vi "test-translation2d.vi"() -> ()   [LabVIEW 2019]
uses:
  <vilib>/Rock Robotics/WPI/ThirdParty/JAS_Junk/TrajLib/Util_CalcDist.vi
  <vilib>/Rock Robotics/WPI/ThirdParty/JAS_Junk/TrajLib/Trajectory_Library.lvlib
panel:
  out "T7 -- y -- 0":dbl
  out "T7 -- X -- 0":dbl
  out "T6 -- dist - 0":dbl
  out "T5 -- norm - 0":dbl
  out "T4 -- y -- 0":dbl
  out "T4 -- X -- 0":dbl
  out "T3 -- y -- 0":dbl
  out "T3 -- X -- 0":dbl
  out "T2 -- y -- 0":dbl
  out "T2 -- X -- 0":dbl
  out "T9 - False":bool
  out "T8 - True":bool
  out "T1 -- y -- 0":dbl
  out "T1 -- X -- 0":dbl
  out "T0 -- y -- 0":dbl
  out "T0 -- X -- 0":dbl
  # "Translation2D Test"
  # "Didn't implement divide"
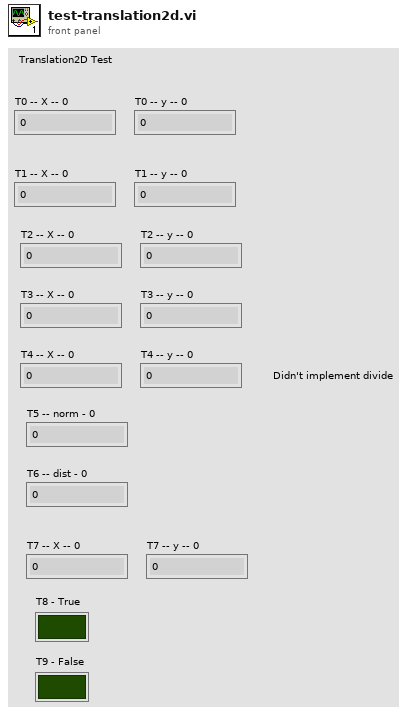
[diagram p1: front panel]
types:
  T1 = typedef "Trajectory_Library.lvlib/TRANSLATION2D.ctl" = cluster{"X":dbl, "Y":dbl}
  T2 = typedef "Trajectory_Library.lvlib/ROTATION2D.ctl" = cluster{"VALUE":dbl, "COS":dbl, "SIN":dbl}
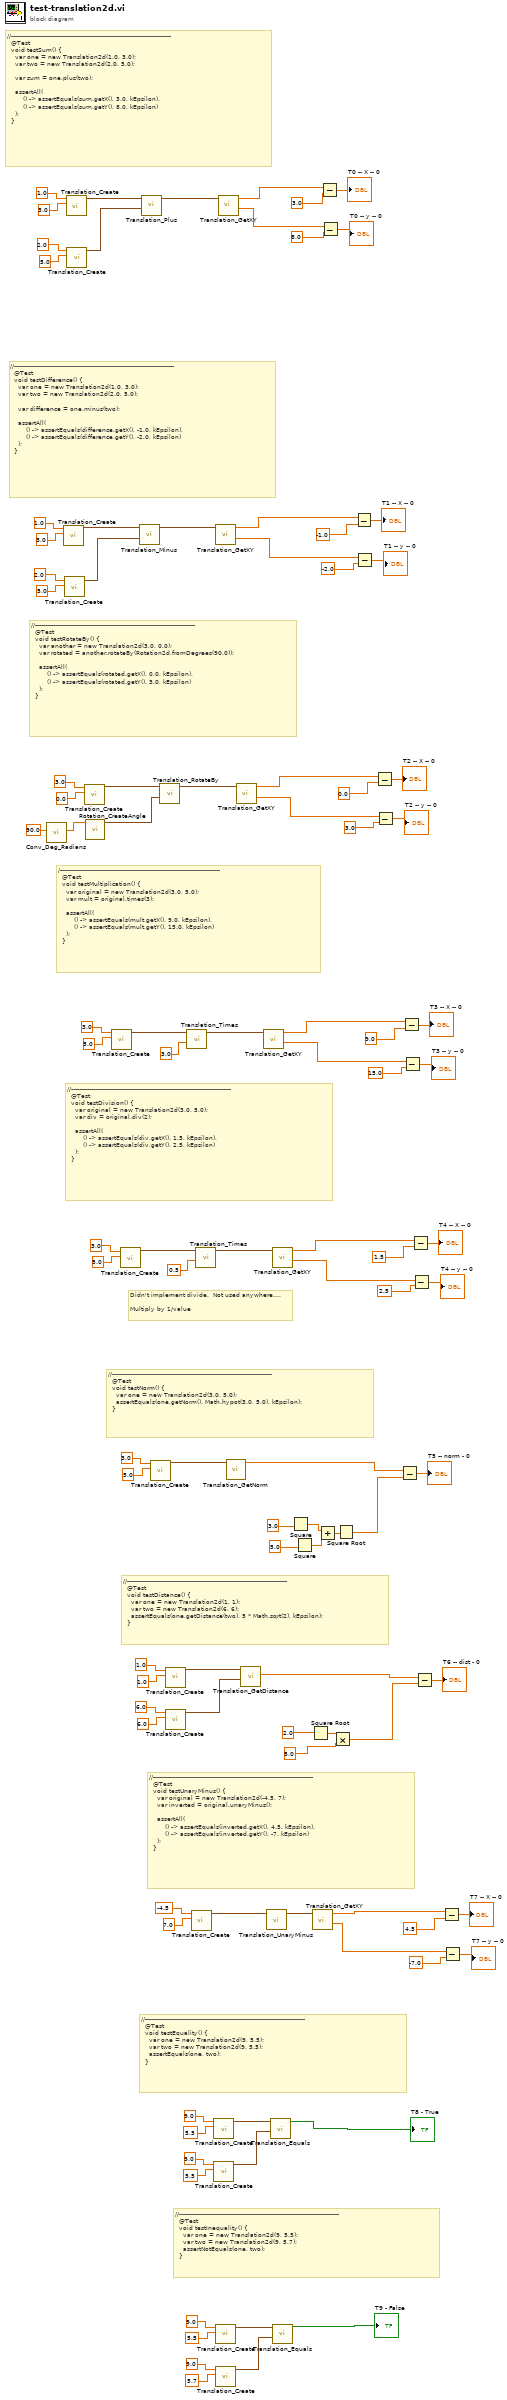
[diagram p0: block diagram]
diagram:
  # "//--------------------------------------------------------------------------------\n  @Test\n  void testInequality() {\n    var one = new Translation2d(9, 5.5);\n    var two = new Translation2d(9, 5.7);\n    assertNotEquals(one, two);\n  }"
  # "//--------------------------------------------------------------------------------\n  @Test\n  void testUnaryMinus() {\n    var original = new Translation2d(-4.5, 7);\n    var inverted = original.unaryMinus();\n\n    assertAll(\n        () -> assertEquals(inverted.getX(), 4.5, kEpsilon),\n        () -> assertEquals(inverted.getY(), -7, kEpsilon)\n    );\n  }"
  # "//--------------------------------------------------------------------------------\n  @Test\n  void testDistance() {\n    var one = new Translation2d(1, 1);\n    var two = new Translation2d(6, 6);\n    assertEquals(one.getDistance(two), 5 * Math.sqrt(2), kEpsilon);\n  }"
  # "//--------------------------------------------------------------------------------\n  @Test\n  void testNorm() {\n    var one = new Translation2d(3.0, 5.0);\n    assertEquals(one.getNorm(), Math.hypot(3.0, 5.0), kEpsilon);\n  }"
  # "Didn't implement divide.  Not used anywhere....\n\nMultiply by 1/value"
  # "//--------------------------------------------------------------------------------\n  @Test\n  void testDivision() {\n    var original = new Translation2d(3.0, 5.0);\n    var div = original.div(2);\n\n    assertAll(\n        () -> assertEquals(div.getX(), 1.5, kEpsilon),\n        () -> assertEquals(div.getY(), 2.5, kEpsilon)\n    );\n  }"
  # "/--------------------------------------------------------------------------------\n  @Test\n  void testMultiplication() {\n    var original = new Translation2d(3.0, 5.0);\n    var mult = original.times(3);\n\n    assertAll(\n        () -> assertEquals(mult.getX(), 9.0, kEpsilon),\n        () -> assertEquals(mult.getY(), 15.0, kEpsilon)\n    );\n  }"
  # "//--------------------------------------------------------------------------------\n  @Test\n  void testRotateBy() {\n    var another = new Translation2d(3.0, 0.0);\n    var rotated = another.rotateBy(Rotation2d.fromDegrees(90.0));\n\n    assertAll(\n        () -> assertEquals(rotated.getX(), 0.0, kEpsilon),\n        () -> assertEquals(rotated.getY(), 3.0, kEpsilon)\n    );\n  }"
  # "//--------------------------------------------------------------------------------\n  @Test\n  void testEquality() {\n    var one = new Translation2d(9, 5.5);\n    var two = new Translation2d(9, 5.5);\n    assertEquals(one, two);\n  }"
  # "//--------------------------------------------------------------------------------\n  @Test\n  void testDifference() {\n    var one = new Translation2d(1.0, 3.0);\n    var two = new Translation2d(2.0, 5.0);\n\n    var difference = one.minus(two);\n\n    assertAll(\n        () -> assertEquals(difference.getX(), -1.0, kEpsilon),\n        () -> assertEquals(difference.getY(), -2.0, kEpsilon)\n    );\n  }"
  # "//--------------------------------------------------------------------------------\n  @Test\n  void testSum() {\n    var one = new Translation2d(1.0, 3.0);\n    var two = new Translation2d(2.0, 5.0);\n\n    var sum = one.plus(two);\n\n    assertAll(\n        () -> assertEquals(sum.getX(), 3.0, kEpsilon),\n        () -> assertEquals(sum.getY(), 8.0, kEpsilon)\n    );\n  }"
  n1 = call <vilib>:"Conv_Deg_Radians.vi"("Degress"=90.0) -> ("Radians"=w72:dbl)  [unwired: 10 in]
  n2 = call <vilib>:"Translation_Create.vi"("Y"=3.0, "X"=1.0) -> ("TRANSLATION"=w88:T1)  [unwired: 9 in]
  n3 = call <vilib>:"Translation_Create.vi"("Y"=5.0, "X"=2.0) -> ("TRANSLATION"=w87:T1)  [unwired: 9 in]
  n4 = call <vilib>:"Translation_Create.vi"("Y"=3.0, "X"=1.0) -> ("TRANSLATION"=w97:T1)  [unwired: 9 in]
  n5 = call <vilib>:"Translation_Create.vi"("Y"=5.0, "X"=2.0) -> ("TRANSLATION"=w96:T1)  [unwired: 9 in]
  n6 = call <vilib>:"Translation_Create.vi"("Y"=0.0, "X"=3.0) -> ("TRANSLATION"=w77:T1)  [unwired: 9 in]
  n7 = call <vilib>:"Rotation_CreateAngle.vi"("Angle"=w72) -> ("ROTATION"=w70:T2)  [unwired: 10 in]
  n8 = call <vilib>:"Translation_Create.vi"("Y"=5.0, "X"=3.0) -> ("TRANSLATION"=w64:T1)  [unwired: 9 in]
  n9 = call <vilib>:"Translation_Create.vi"("Y"=5.0, "X"=3.0) -> ("TRANSLATION"=w53:T1)  [unwired: 9 in]
  n10 = call <vilib>:"Translation_Minus.vi"("other Translation"=w87, "In Translation"=w88) -> ("Out Translation"=w86:T1)  [unwired: 9 in]
  n11 = call <vilib>:"Translation_Plus.vi"("other Translation"=w96, "In Translation"=w97) -> ("Out Translation"=w95:T1)  [unwired: 9 in]
  n12 = call <vilib>:"Translation_Create.vi"("Y"=5.0, "X"=3.0) -> ("TRANSLATION"=w44:T1)  [unwired: 9 in]
  n13 = call <vilib>:"Translation_RotateBy.vi"("other Rotation"=w70, "In Translation"=w77) -> ("Out Translation"=w76:T1)  [unwired: 9 in]
  n14 = call <vilib>:"Translation_Create.vi"("Y"=1.0, "X"=1.0) -> ("TRANSLATION"=w33:T1)  [unwired: 9 in]
  n15 = call <vilib>:"Translation_Create.vi"("Y"=6.0, "X"=6.0) -> ("TRANSLATION"=w29:T1)  [unwired: 9 in]
  n16 = call <vilib>:"Translation_Times.vi"("Scalar"=3.0, "In Translation"=w64) -> ("Out Translation"=w63:T1)  [unwired: 9 in]
  n17 = call <vilib>:"Translation_Create.vi"("Y"=7.0, "X"=-4.5) -> ("TRANSLATION"=w22:T1)  [unwired: 9 in]
  n18 = call <vilib>:"Translation_Times.vi"("Scalar"=0.5, "In Translation"=w53) -> ("Out Translation"=w52:T1)  [unwired: 9 in]
  n19 = call <vilib>:"Translation_Create.vi"("Y"=5.5, "X"=9.0) -> ("TRANSLATION"=w9:T1)  [unwired: 9 in]
  n20 = call <vilib>:"Translation_Create.vi"("Y"=5.5, "X"=9.0) -> ("TRANSLATION"=w8:T1)  [unwired: 9 in]
  n21 = call <vilib>:"Translation_GetXY.vi"("In Translation"=w86) -> ("Y"=w84:dbl, "X"=w85:dbl)  [unwired: 9 in]
  n22 = call <vilib>:"Translation_Create.vi"("Y"=5.5, "X"=9.0) -> ("TRANSLATION"=w3:T1)  [unwired: 9 in]
  n23 = call <vilib>:"Translation_Create.vi"("Y"=5.7, "X"=9.0) -> ("TRANSLATION"=w2:T1)  [unwired: 9 in]
  n24 = call <vilib>:"Translation_GetXY.vi"("In Translation"=w95) -> ("Y"=w101:dbl, "X"=w102:dbl)  [unwired: 9 in]
  n25 = call <vilib>:"Translation_GetNorm.vi"("In Translation"=w44) -> ("Norm"=w38:dbl)  [unwired: 10 in]
  n26 = call <vilib>:"Translation_GetXY.vi"("In Translation"=w76) -> ("Y"=w74:dbl, "X"=w75:dbl)  [unwired: 9 in]
  n27 = call <vilib>:"Translation_GetDistance.vi"("other Translation"=w29, "In Translation"=w33) -> ("Distance"=w32:dbl)  [unwired: 9 in]
  n28 = call <vilib>:"Translation_GetXY.vi"("In Translation"=w63) -> ("Y"=w61:dbl, "X"=w62:dbl)  [unwired: 9 in]
  n29 = call <vilib>:"Translation_UnaryMinus.vi"("In Translation"=w22) -> ("Out Translation"=w17:T1)  [unwired: 10 in]
  n30 = call <vilib>:"Translation_Equals.vi"("other Translation"=w8, "In Translation"=w9) -> ("Equals"=→"T8 - True":bool)  [unwired: 9 in]
  n31 = call <vilib>:"Translation_GetXY.vi"("In Translation"=w52) -> ("Y"=w50:dbl, "X"=w51:dbl)  [unwired: 9 in]
  n32 = call <vilib>:"Translation_Equals.vi"("other Translation"=w2, "In Translation"=w3) -> ("Equals"=→"T9 - False":bool)  [unwired: 9 in]
  n33 = Square(x=3.0 ("X")) -> (x^2=w40:dbl)
  n34 = Square(x=5.0 ("X")) -> (x^2=w39:dbl)
  n35 = Square Root(x=2.0 ("X")) -> (sqrt(x)=w27:dbl)
  n36 = call <vilib>:"Translation_GetXY.vi"("In Translation"=w17) -> ("Y"=w15:dbl, "X"=w16:dbl)  [unwired: 9 in]
  n37 = Add(x=w40, y=w39) -> (x+y=w41:dbl)
  n38 = Subtract(x=w102, y=3.0) -> (x-y=→"T0 -- X -- 0":dbl)
  n39 = Subtract(x=w101, y=8.0) -> (x-y=→"T0 -- y -- 0":dbl)
  n40 = Multiply(x=w27, y=5.0 ("X")) -> (x*y=w25:dbl)
  n41 = Square Root(x=w41) -> (sqrt(x)=w37:dbl)
  n42 = Subtract(x=w85, y=-1.0 ("x")) -> (x-y=→"T1 -- X -- 0":dbl)
  n43 = Subtract(x=w84, y=-2.0) -> (x-y=→"T1 -- y -- 0":dbl)
  n44 = Subtract(x=w75, y=0.0 ("x")) -> (x-y=→"T2 -- X -- 0":dbl)
  n45 = Subtract(x=w74, y=3.0) -> (x-y=→"T2 -- y -- 0":dbl)
  n46 = Subtract(x=w38, y=w37) -> (x-y=→"T5 -- norm - 0":dbl)
  n47 = Subtract(x=w62, y=9.0 ("x")) -> (x-y=→"T3 -- X -- 0":dbl)
  n48 = Subtract(x=w61, y=15.0) -> (x-y=→"T3 -- y -- 0":dbl)
  n49 = Subtract(x=w51, y=1.5 ("x")) -> (x-y=→"T4 -- X -- 0":dbl)
  n50 = Subtract(x=w50, y=2.5) -> (x-y=→"T4 -- y -- 0":dbl)
  n51 = Subtract(x=w32, y=w25) -> (x-y=→"T6 -- dist - 0":dbl)
  n52 = Subtract(x=w16, y=4.5 ("x")) -> (x-y=→"T7 -- X -- 0":dbl)
  n53 = Subtract(x=w15, y=-7.0) -> (x-y=→"T7 -- y -- 0":dbl)
